vi "Read Directory to delete.vi"(8 "error in (no error)":errorcluster, 11 "[Test Case] Create directory in":refnum<class "[Test Case] Create directory.lvclass">) -> (0 "error out":errorcluster, 2 "Directory to delete":string, 3 "[Test Case] Create directory out":refnum<class "[Test Case] Create directory.lvclass">)   [LabVIEW 2015, in "Tests.lvlib" / "[Test Case] Create directory.lvclass"]
uses:
  [Test Case] Create directory.lvclass
  [Test Case] Create directory.lvclass/[Test Case] Create directory.ctl
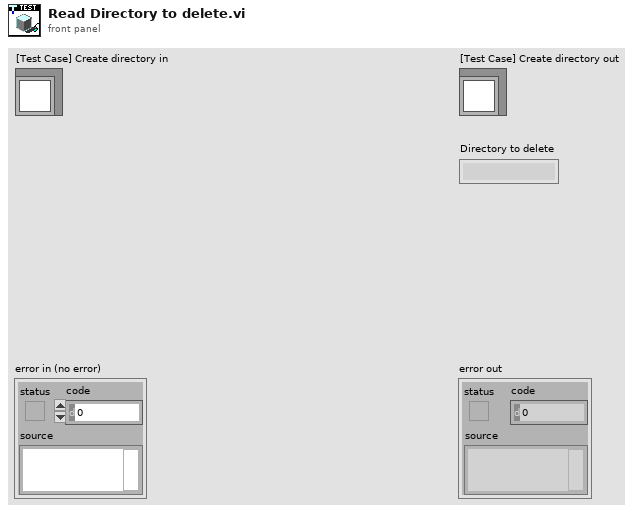
[diagram p1: front panel]
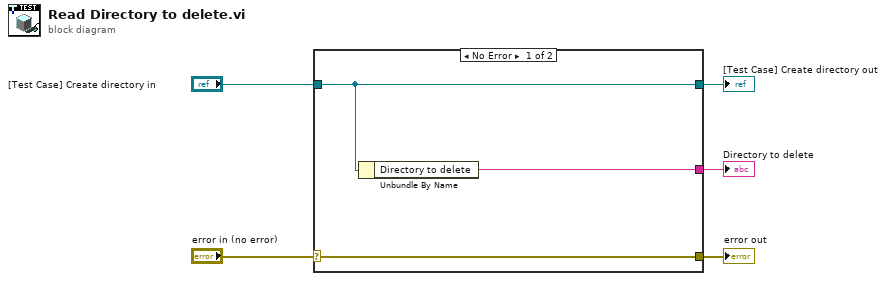
[diagram p0: block diagram]
diagram:
  n1 = case shown="No Error" "error in (no error)" {
    selector: "error in (no error)" -> [w8 w9]
    tunnel: [w8 w9] -> w4
    tunnel: [w7 w10] -> w2
    tunnel: "[Test Case] Create directory in" -> [w7 w10]
    tunnel: [w6 _] -> w1
    frame No Error {
      n2 = Unbundle By Name(w7) -> ("Directory to delete"=w6:string)
    }
    frame Error {
    }
  }
  "error out" <- w4
  "[Test Case] Create directory out" <- w2
  "Directory to delete" <- w1
